vi "ProducerConsumerEvents PC Host.vi"() -> ()   [LabVIEW 2015]
uses:
  <vilib>/rvi/interface/nirviOpenFPGA/nirviOpenFPGA.xnode
  <vilib>/rvi/interface/nirviMethod/nirviMethod.xnode
  <vilib>/FPGAPlugInAG/Dynamic/niLvFpga_Reset_Dynamic.vi
  <vilib>/FPGAPlugInAG/Dynamic/niLvFpga_Run_Dynamic.vi
  Globals.vi
  <vilib>/rvi/interface/nirviReadWriteControl/nirviReadWriteControl.xnode
  FPGA Host.vi
  <vilib>/rvi/interface/Simulation/niFpgaSimulationCallBeginRW.vi
  <vilib>/rvi/errors/niLvFpgaAdjustHostInterfaceError.vi
  <vilib>/rvi/interface/RandomDataEmulation/nirviRandomDataOpen.vi
  <vilib>/rvi/interface/common/niFpgaCacheSessionInfoDynamic.vi
  <vilib>/FPGAPlugInAG/Dynamic/niLvFpga_WriteFifo_Dynamic.vi
  <vilib>/rvi/errors/niLvFpgaMergeErrorWithErrorCode.vi
panel:
  out "error out":errorcluster
  out "Waveform Exist":bool
  in  "Resolution":u16(ring)=512 items=["2048*2048"=2048, "1024*1024"=1024, "512*512"=512, "256*256"=256]
  out "Events with Data":i32
  out "Waveform to FIFO done":bool
  out "大小":i32[](array[numeric])
  out "数组":u16[][](array[numeric])
  out "WaveXY":u16[](array[numeric])
  out "WaveY":u16[](graph)
  in  "Galvo Waveform data Y":path=path "C:/Users/hppc/Desktop/OpenScan/New Structure/waveY.txt"
  in  "Initialize":bool caption="停止"
  in  "Start Scanning":bool caption="元素入队列"
  out "WaveX":u16[](graph)
  out "Waveform Points":i32=5120
  in  "Galvo Waveform data X":path=path "C:/Users/hppc/Desktop/OpenScan/New Structure/waveX.txt"
  in  "Load Waveform":bool caption="元素入队列"
  in  "stop":bool caption="停止"
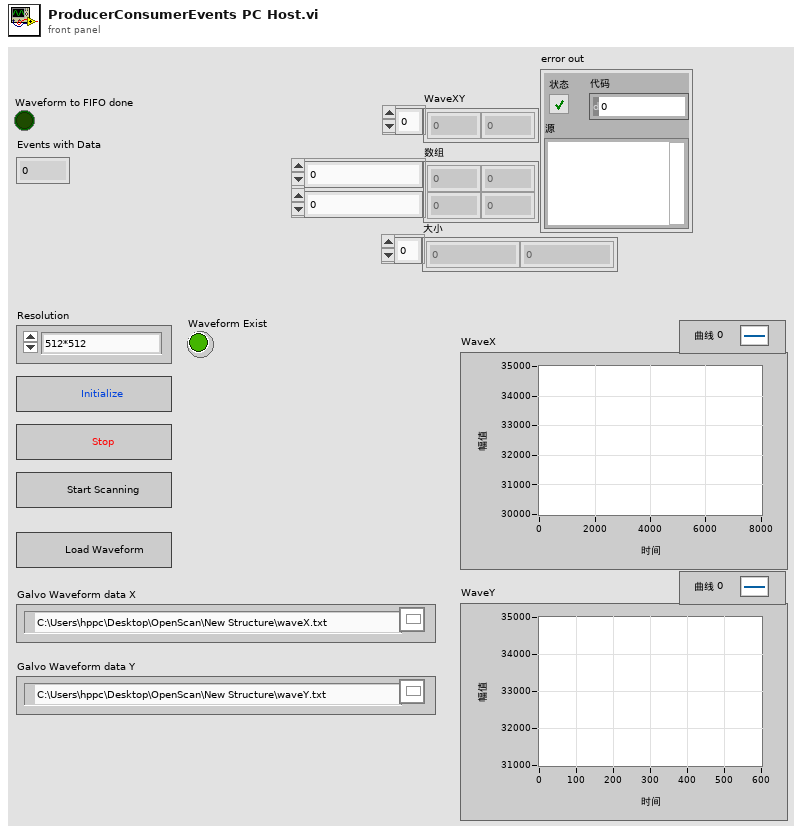
[diagram p1: front panel]
types:
  T1 = enum16{"Load Waveform", "Start Scanning", "Save Image", "Stop"}
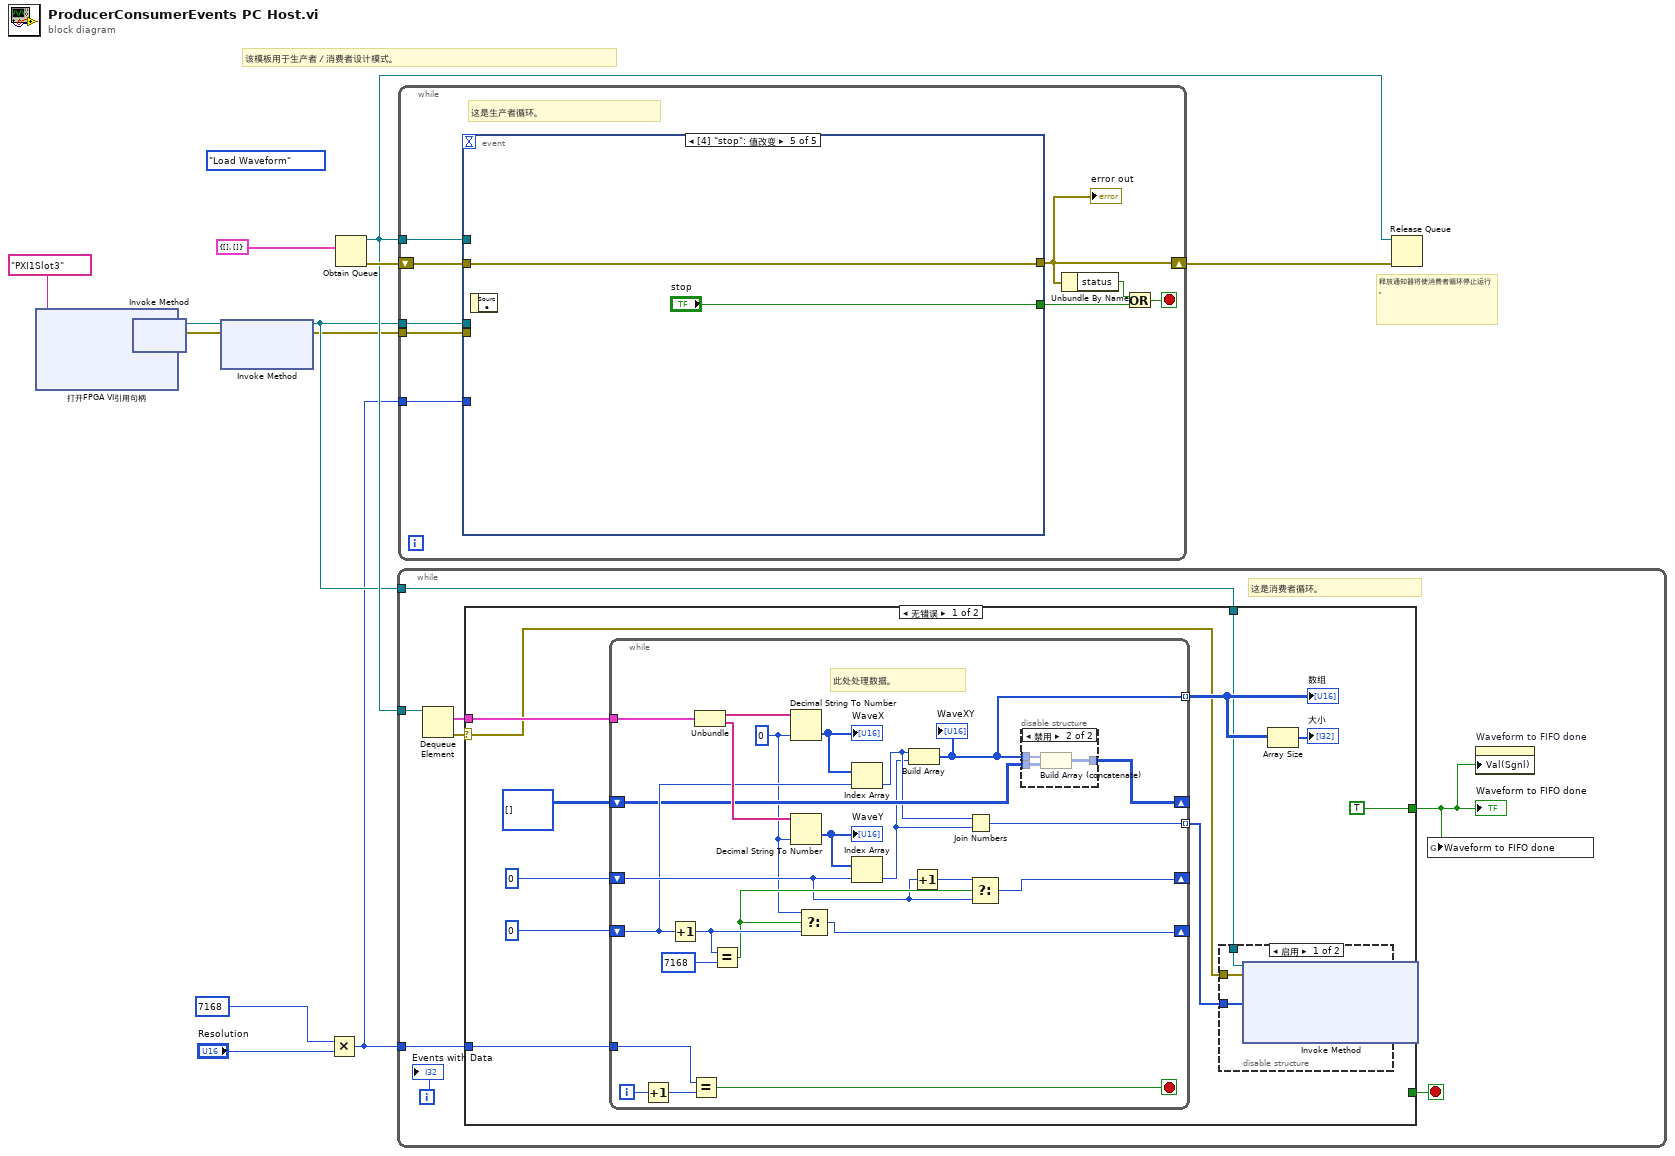
[diagram p0: block diagram]
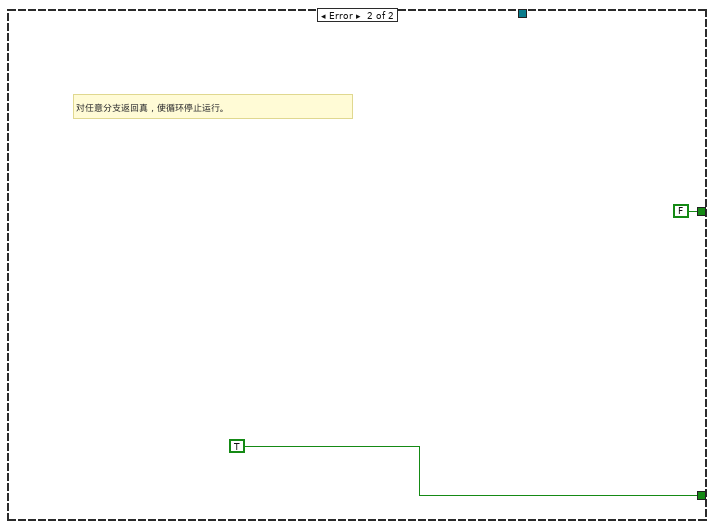
[diagram p4: hidden frame]
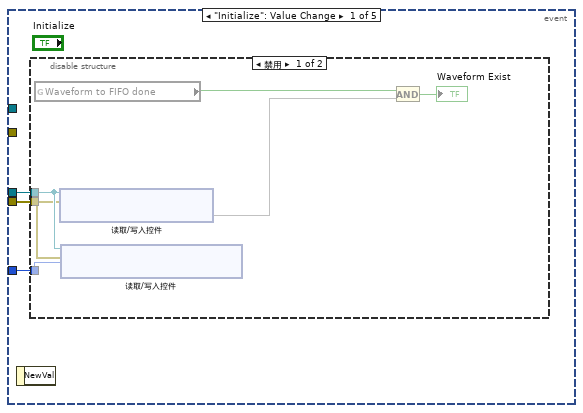
[diagram p5: hidden frame]
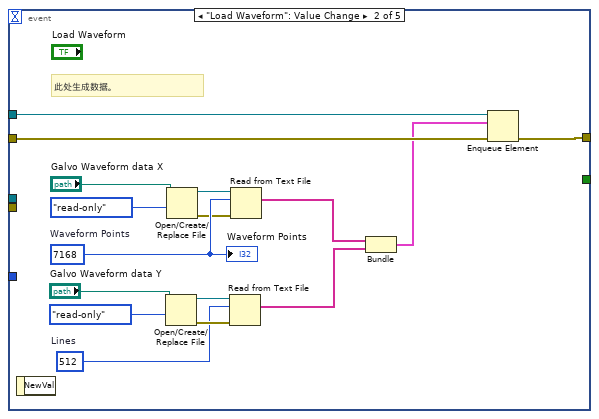
[diagram p7: hidden frame]
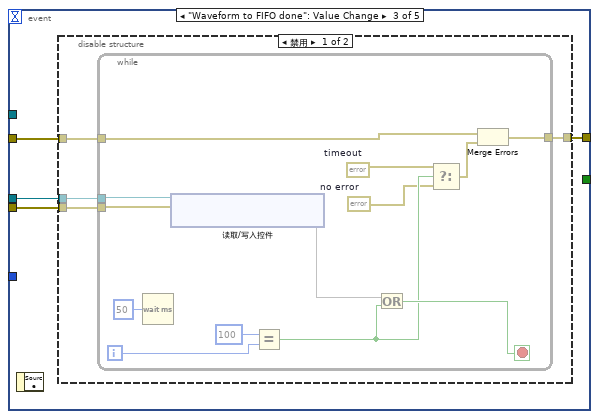
[diagram p8: hidden frame]
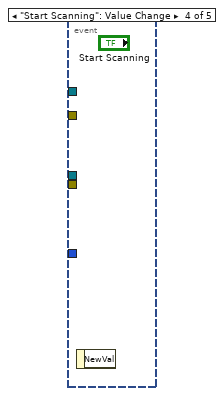
[diagram p10: hidden frame]
diagram:
  (unwired) T1."Load Waveform"
  # "释放通知器将使消费者循环停止运行。"
  # "该模板用于生产者／消费者设计模式。"
  n1 = xnode "打开FPGA VI引用句柄"("资源名称"=tag "PXI1Slot3") -> ("FPGA VI引用输出"=w9:refnum<k20>, "错误输出"=w8:errorcluster)  [unwired: 1 in]
  n2 = xnode "Invoke Method"("FPGA VI引用输入"=w9, "错误输入"=w8) -> ("FPGA VI引用输出"=w7:refnum<k20>, "错误输出"=w6:errorcluster)
  n3 = xnode "Invoke Method"("FPGA VI引用输入"=w7, "错误输入"=w6) -> ("FPGA VI引用输出"=w5:refnum<k20>, "错误输出"=w4:errorcluster)  [unwired: 1 in]
  n4 = Multiply(x=7168, y="Resolution") -> (x*y=w1:i32)
  n5 = Obtain Queue(element data type=cluster{string[], string[]} {[], []} ("输出簇")) -> (queue out=w12:refnum<queue>, error out=w14:errorcluster)  [unwired: 4 in, 1 out]
  n6 = while {
    tunnel: w12 -> [w22]
    tunnel: w1 -> [w18]
    tunnel: w5 -> [w17]
    i -> [w16]
    stop <- w20 stop-if-true
    # "这是消费者循环。"
    n7 = Dequeue Element(queue=w22) -> (element=w19:cluster{string[], string[]}, error out=w21:errorcluster)  [unwired: 2 in, 2 out]
    n8 = case shown="无错误" w21 {
      selector: w21 -> [w25 _]
      tunnel: [_ TRUE] -> w20
      tunnel: w19 -> [w33 _]
      tunnel: w18 -> [w29 _]
      tunnel: w17 -> [w26 _]
      tunnel: [TRUE FALSE] -> w15
      frame No Error {
        n9 = while {
          tunnel: w33 -> [w60]
          shift-right: [w50] -> _
          shift-left: 0 ("索引") -> [w51]
          shift-right: [w54] -> _
          shift-left: 0 ("索引") -> [w48]
          shift-right: [w42] -> _
          shift-left: u16[][] [] ("添加的数组") -> [w47]
          tunnel: w29 -> [w44]
          tunnel: [w40] -> w27 mode=indexing
          tunnel: [w37] -> w24 mode=indexing
          i -> [w45]
          stop <- w46 stop-if-true
          w41 = u16 0 ("默认(0 I32)")
          # "此处处理数据。"
          n10 = Increment(x=w45) -> (x+1=w43:i32)
          n11 = Increment(x=w48) -> (x+1=w55:i32)
          n12 = Equal?(x=w44, y=w43) -> (x = y?=w46:bool)
          n13 = Unbundle(w60) -> (w59:string[], w58:string[])
          n14 = Equal?(x=w55, y=7168) -> (x = y?=w53:bool)
          n15 = Decimal String To Number(string=w59, default (0L)=w41) -> (number=w49:u16[])  [unwired: 1 in, 1 out]
          "WaveX" <- w49
          n16 = Decimal String To Number(string=w58, default (0L)=w41) -> (number=w57:u16[])  [unwired: 1 in, 1 out]
          "WaveY" <- w57
          n17 = Select(t=w41, s=w53, f=w55) -> (s? t:f=w54:i32)
          n18 = Index Array(array=w49, index=w48) -> (element=w39:u16)
          n19 = Index Array(array=w57, index=w51) -> (element=w38:u16)
          n20 = Build Array(w39, w38) -> (w40:u16[])
          "WaveXY" <- w40
          n21 = Increment(x=w51) -> (x+1=w52:i32)
          n22 = Join Numbers(hi=w39, lo=w38) -> ((hi.lo)=w37:u32)
          n23 = Select(t=w52, s=w53, f=w51) -> (s? t:f=w50:i32)
          n24 = disable-structure shown="禁用" {
            disable-tunnel: w47 -> [_ w63]
            disable-tunnel: [_ w62] -> w42
            disable-tunnel: w40 -> [_ w61]
            frame Enabled {
            }
            frame Disabled {
              n25 = Build Array (concatenate)(w61, w63) -> (w62:u16[][])
            }
          }
        }
        "数组" <- w27
        n26 = disable-structure shown="启用" {
          disable-tunnel: w26 -> [w36 _]
          disable-tunnel: w25 -> [w35 _]
          disable-tunnel: w24 -> [w34 _]
          frame Enabled {
            n27 = xnode "Invoke Method"("FPGA VI引用输入"=w36, "错误输入"=w35, "Data"=w34) -> ()  [unwired: 1 in, 3 out]
          }
          frame Disabled {
          }
        }
        n28 = Array Size(array=w27) -> (size(s)=→"大小":i32[])
      }
      frame Error {
        # "对任意分支返回真，使循环停止运行。"
      }
    }
    "Waveform to FIFO done" <- w15
    n29 = global write "Globals.vi" "Waveform to FIFO done"(w15) -> ()
    n30 = property on="Waveform to FIFO done" class="Bool (严格)"("Val(Sgnl)"=w15) -> ()  [unwired: 2 in, 2 out]
    "Events with Data" <- w16
  }
  n31 = while {
    shift-right: [w70] -> w13
    shift-left: w14 -> [w73]
    tunnel: w12 -> [w74]
    tunnel: w4 -> [w67]
    tunnel: w1 -> [w66]
    tunnel: w5 -> [w68]
    stop <- w71 stop-if-true
    # "这是生产者循环。"
    n32 = event shown="[4] \"stop\": 值改变" {
      selector: _ -> [_ _ _ _ _]
      dyn-events: _ -> [_ _ _ _ _]
      timeout: _ -> [_ _ _ _ _]
      tunnel: w74 -> [_ w99 _ _ _]
      tunnel: w73 -> [_ w98 w100 _ w121]
      tunnel: [_ w97 w101 _ w121] -> w70
      tunnel: [_ _ _ _ "stop"] -> w72
      tunnel: w68 -> [w77 _ w103 _ _]
      tunnel: w67 -> [w76 _ w102 _ _]
      tunnel: w66 -> [w75 _ _ _ _]
      event "Initialize": Value Change {
        n33 = event-data() -> ()  [unwired: 1 in, 1 out]
        n34 = disable-structure shown="禁用" {
          disable-tunnel: w77 -> [w80 _]
          disable-tunnel: w76 -> [w79 _]
          disable-tunnel: w75 -> [w78 _]
          frame Disabled {
            n35 = global read "Globals.vi" "Waveform to FIFO done"() -> (w82:bool)
            n36 = xnode "读取/写入控件"("FPGA VI引用输入"=w80, "错误输入"=w79) -> ("Waveform DRAM done"=w83)  [unwired: 2 out]
            n37 = xnode "读取/写入控件"("FPGA VI引用输入"=w80, "错误输入"=w79, "Total Waveform data points"=w78) -> ()  [unwired: 2 out]
            n38 = And(x=w82, y=w83) -> (x .and. y?=→"Waveform Exist":bool)
          }
          frame Enabled {
          }
        }
      }
      event "Load Waveform": Value Change {
        w90 = 512  # Lines
        w93 = 7168  # Waveform Points
        # "此处生成数据。"
        n39 = event-data() -> ()  [unwired: 1 in, 1 out]
        n40 = Open/Create/Replace File(file path (use dialog)="Galvo Waveform data Y", access (0:read/write)=enum16{"read/write", "read-only", "write-only"}."read-only" ("权限(0:read/write)")) -> (refnum out=w89:refnum<file>, error out=w91:errorcluster)  [unwired: 4 in, 1 out]
        n41 = Open/Create/Replace File(file path (use dialog)="Galvo Waveform data X", access (0:read/write)=enum16{"read/write", "read-only", "write-only"}."read-only" ("权限(0:read/write)")) -> (refnum out=w94:refnum<file>, error out=w92:errorcluster)  [unwired: 4 in, 1 out]
        n42 = Read from Text File(file (use dialog)=w89, count=w90, error in=w91) -> (text=w85:string[])  [unwired: 1 in, 3 out]
        n43 = Read from Text File(file (use dialog)=w94, count=w93, error in=w92) -> (text=w86:string[])  [unwired: 1 in, 3 out]
        n44 = Bundle(w86, w85) -> (w84:cluster{string[], string[]})  [unwired: 1 in]
        n45 = Enqueue Element(queue=w99, element=w84, error in (no error)=w98) -> (error out=w97:errorcluster)  [unwired: 1 in, 2 out]
        "Waveform Points" <- w93
      }
      event "Waveform to FIFO done": Value Change {
        n46 = event-data() -> ()  [unwired: 1 in, 1 out]
        n47 = disable-structure shown="禁用" {
          disable-tunnel: w103 -> [w107 _]
          disable-tunnel: w102 -> [w106 _]
          disable-tunnel: [w105 _] -> w101
          disable-tunnel: w100 -> [w104 _]
          frame Disabled {
            n48 = while {
              tunnel: w107 -> [w120]
              tunnel: w106 -> [w119]
              tunnel: [w113] -> w105
              tunnel: w104 -> [w112]
              i -> [w117]
              stop <- w114 stop-if-true
              w109 = errorcluster {"status"=FALSE, "code"=0, "source"=""}  # no error
              w110 = errorcluster {"status"=TRUE, "code"=0, "source"="Write Waveform DRAM timeout"}  # timeout
              n49 = Wait (ms)(milliseconds to wait=u32 50 ("等待时间（毫秒）")) -> ()  [unwired: 1 out]
              n50 = xnode "读取/写入控件"("FPGA VI引用输入"=w120, "错误输入"=w119) -> ("Waveform DRAM done"=w115)  [unwired: 2 out]
              n51 = Equal?(x=100, y=w117) -> (x = y?=w111:bool)
              n52 = Or(x=w115, y=w111) -> (x .or. y?=w114:bool)
              n53 = Select(t=w110, s=w111, f=w109) -> (s? t:f=w108:errorcluster)
              n54 = Merge Errors(w112, w108) -> (w113:errorcluster)
            }
          }
          frame Enabled {
          }
        }
      }
      event "Start Scanning": Value Change {
        n55 = event-data() -> ()  [unwired: 1 in, 1 out]
      }
      event "stop": Value Change {
        n56 = event-data() -> ()  [unwired: 1 in, 1 out]
      }
    }
    "error out" <- w70
    n57 = Unbundle By Name(w70) -> ("status"=w69:bool)
    n58 = Or(x=w69, y=w72) -> (x .or. y?=w71:bool)
  }
  n59 = Release Queue(queue=w12, error in (no error)=w13) -> ()  [unwired: 1 in, 3 out]
